vi "Spex Goto.vi"(7 "Moving Ref":refnum<vi>, 8 "error in":errorcluster, 9 "Lambda Ref":refnum<vi>, 10 "Wl(nm)":dbl caption="Wavelenght(nm)" format="%#.3g", 11 "Port":refnum<visa-resource-name>="COM1" caption="Com Port") -> (0 "error out":errorcluster, 3 "SpexOut":string caption="Spex Output")   [LabVIEW 2010]
uses:
  <vilib>/Instr/_visa.llb/VISA Configure Serial Port (Instr).vi
  <userlib>/GenProg/WritebyRefBool.vi
  <userlib>/GenProg/WritebyRefNum.vi
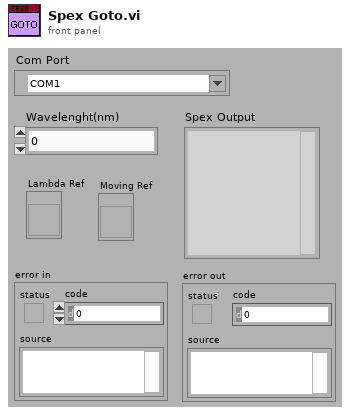
[diagram p1: front panel]
types:
  T1 = enum16{"Send Par", "Wait Answer", "Send Com", "Wait End", "Error"}
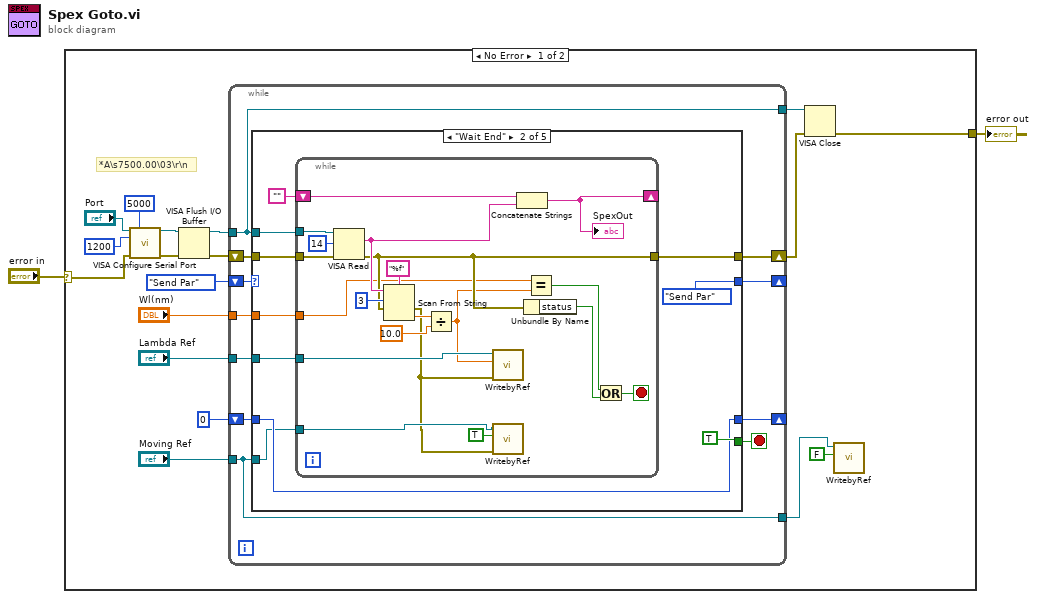
[diagram p0: block diagram]
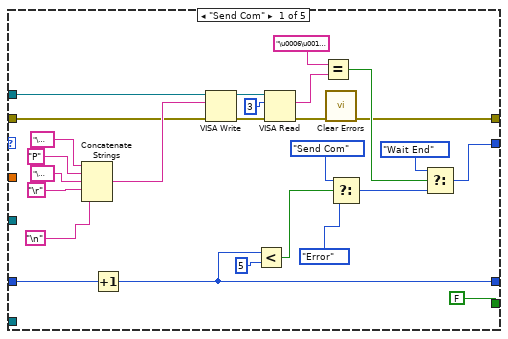
[diagram p2: hidden frame]
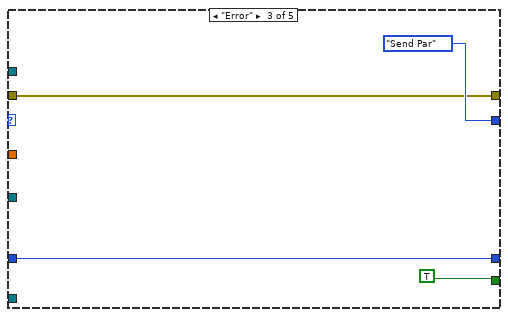
[diagram p3: hidden frame]
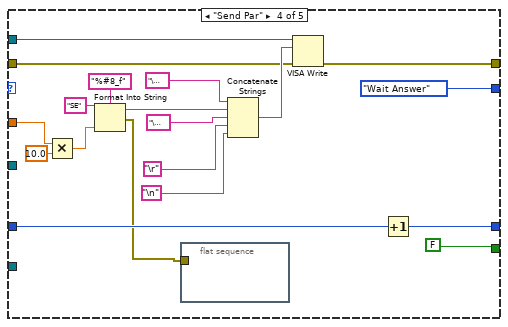
[diagram p4: hidden frame]
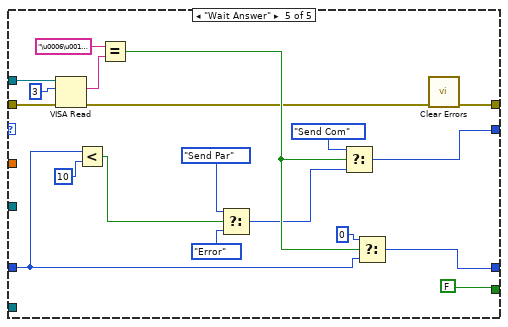
[diagram p5: hidden frame]
diagram:
  n1 = case shown="No Error" "error in" {
    selector: "error in" -> [w8 w130]
    tunnel: [w9 w130] -> w2
    frame No Error {
      # "*A\\s7500.00\\03\\r\\n"
      n2 = call-poly "VISA Configure Serial Port"("VISA resource name"="Port", "timeout (10sec)"=u32 5000, "baud rate (9600)"=u32 1200, "error in (no error)"=w8) -> ("VISA resource name out"=w17:refnum<visa-resource-name>, "error out"=w18:errorcluster)  [unwired: 10 in]
      n3 = VISA Flush I/O Buffer(VISA resource name=w17, error in (no error)=w18) -> (VISA resource name out=w16:refnum<visa-resource-name>, error out=w11:errorcluster)  [unwired: 1 in]
      n4 = while {
        shift-right: [w28] -> _
        shift-left: T1."Send Par" -> [w31]
        tunnel: w16 -> [w26]
        shift-right: [w29] -> w10
        shift-left: w11 -> [w30]
        tunnel: [w26] -> w15
        shift-right: [w24] -> _
        shift-left: 0 -> [w25]
        tunnel: "Lambda Ref" -> [w23]
        tunnel: "Wl(nm)" -> [w22]
        tunnel: "Moving Ref" -> [w21]
        tunnel: [w21] -> w3
        stop <- w27 stop-if-true
        n5 = case shown="\"Wait End\"" w31 {
          tunnel: w26 -> [w32 w66 _ w105 w125]
          tunnel: w30 -> [w33 w65 w88 w104 w114]
          tunnel: [w36 w64 w88 w103 w112] -> w29
          tunnel: [w47 T1."Send Par" T1."Send Par" T1."Wait Answer" w127] -> w28
          tunnel: [FALSE TRUE TRUE FALSE FALSE] -> w27
          tunnel: w25 -> [w40 w60 w89 w97 w111]
          tunnel: [w37 w60 w89 w96 w115] -> w24
          tunnel: w23 -> [_ w59 _ _ _]
          tunnel: w22 -> [_ w61 _ w95 _]
          tunnel: w21 -> [_ w58 _ _ _]
          frame "Send Com" {
            n6 = Concatenate Strings("\u0018" ("string"), "P" ("string"), "\u0003" ("string"), "\r", "\n") -> (w52:string)
            n7 = Increment(x=w40) -> (x+1=w37:i32)
            n8 = VISA Write(VISA resource name=w32, write buffer=w52, error in (no error)=w33) -> (VISA resource name out=w48:refnum<visa-resource-name>, error out=w49:errorcluster)  [unwired: 1 out]
            n9 = Less?(x=w37, y=5) -> (x < y?=w38:bool)
            n10 = VISA Read(VISA resource name=w48, byte count=u32 3, error in (no error)=w49) -> (read buffer=w44:string, error out=w35:errorcluster)  [unwired: 2 out]
            n11 = Equal?(x="\u0006\u0018\u0018", y=w44) -> (x = y?=w45:bool)
            n12 = call <vilib>:"Clear Errors.vi"("error in (no error)"=w35) -> ("error out"=w36:errorcluster)  [unwired: 6 in]
            n13 = Select(t=T1."Send Com" ("f"), s=w38, f=T1."Error") -> (s? t:f=w41:T1)
            n14 = Select(t=T1."Wait End", s=w45, f=w41) -> (s? t:f=w47:T1)
          }
          frame "Wait End" {
            n15 = while {
              tunnel: w66 -> [w81]
              tunnel: w65 -> [w86]
              tunnel: [w74] -> w64
              shift-right: [w80] -> _
              shift-left: "" -> [w82]
              tunnel: w59 -> [w70]
              tunnel: w61 -> [w73]
              tunnel: w58 -> [w72]
              stop <- w84 stop-if-true
              n16 = VISA Read(VISA resource name=w81, byte count=u32 14, error in (no error)=w86) -> (read buffer=w76:string, error out=w74:errorcluster)  [unwired: 2 out]
              n17 = Scan From String(format string="%f", input string=w76, initial scan location=u32 3, error in=w74) -> (error out=w68:errorcluster, output 1=w78:dbl)  [unwired: 1 in, 2 out]
              n18 = Divide(x=w78, y=10.0) -> (x/y=w69:dbl)
              n19 = call-poly <userlib>:"WritebyRef.vi"("error in"=w68, "Valeur"=w69, "Control Ref"=w70) -> ()  [unwired: 8 in, 1 out]
              n20 = call-poly <userlib>:"WritebyRef.vi"("error in"=w68, "Valeur"=TRUE, "Control Ref"=w72) -> ()  [unwired: 8 in, 1 out]
              n21 = Concatenate Strings(w82, w76) -> (w80:string)
              "SpexOut" <- w80
              n22 = Unbundle By Name(w74) -> ("status"=w83:bool)
              n23 = Equal?(x=w73, y=w69) -> (x = y?=w85:bool)
              n24 = Or(x=w85, y=w83) -> (x .or. y?=w84:bool)
            }
          }
          frame "Error" {
          }
          frame "Send Par" {
            n25 = Multiply(x=w95, y=10.0) -> (x*y=w94:dbl)
            n26 = Format Into String(format string="%#8_f", initial string="SE", w94) -> (resulting string=w98:string, error out=w92:errorcluster)  [unwired: 1 in]
            n27 = flat-sequence {
              tunnel: w92 -> [_]
              frame #0 {
              }
            }
            n28 = Concatenate Strings("\u0002" ("string"), w98, "\u0003" ("string"), "\r", "\n") -> (w106:string)
            n29 = VISA Write(VISA resource name=w105, write buffer=w106, error in (no error)=w104) -> (error out=w103:errorcluster)  [unwired: 2 out]
            n30 = Increment(x=w97) -> (x+1=w96:i32)
          }
          frame "Wait Answer" {
            n31 = VISA Read(VISA resource name=w125, byte count=u32 3, error in (no error)=w114) -> (read buffer=w123:string, error out=w113:errorcluster)  [unwired: 2 out]
            n32 = Less?(x=w111, y=10) -> (x < y?=w117:bool)
            n33 = Equal?(x="\u0006\u0018\u0018", y=w123) -> (x = y?=w121:bool)
            n34 = Select(t=T1."Send Par", s=w117, f=T1."Error") -> (s? t:f=w116:T1)
            n35 = Select(t=T1."Send Com", s=w121, f=w116) -> (s? t:f=w127:T1)
            n36 = Select(t=0, s=w121, f=w111) -> (s? t:f=w115:i32)
            n37 = call <vilib>:"Clear Errors.vi"("error in (no error)"=w113) -> ("error out"=w112:errorcluster)  [unwired: 6 in]
          }
        }
      }
      n38 = VISA Close(VISA resource name=w15, error in (no error)=w10) -> (error out=w9:errorcluster)
      n39 = call-poly <userlib>:"WritebyRef.vi"("Valeur"=FALSE, "Control Ref"=w3) -> ()  [unwired: 9 in, 1 out]
    }
    frame Error {
    }
  }
  "error out" <- w2
